vi "Get Queue Ref.vi"(6 "Command":T1=enum."Obtain", 8 "Error In":errorcluster, 11 "Call Chain Index (2)":i32=2) -> (0 "Error Out":errorcluster, 3 "Queue Out":T2)   [LabVIEW 2014, in "SLL QSM.lvlib"]
doc: "Create/Obtain/Delete Queue Reference based on the VI Instance Name. \n\nThe input to the call chain determines the VI for which the Queue Reference need to be obtained."
uses:
  SLL QSM.lvlib
  Typedefs/Queue Reference.ctl
  Typedefs/Queue Type.ctl
  Typedefs/Queue Reference Command.ctl
  Typedefs/Variant LUT Command.ctl
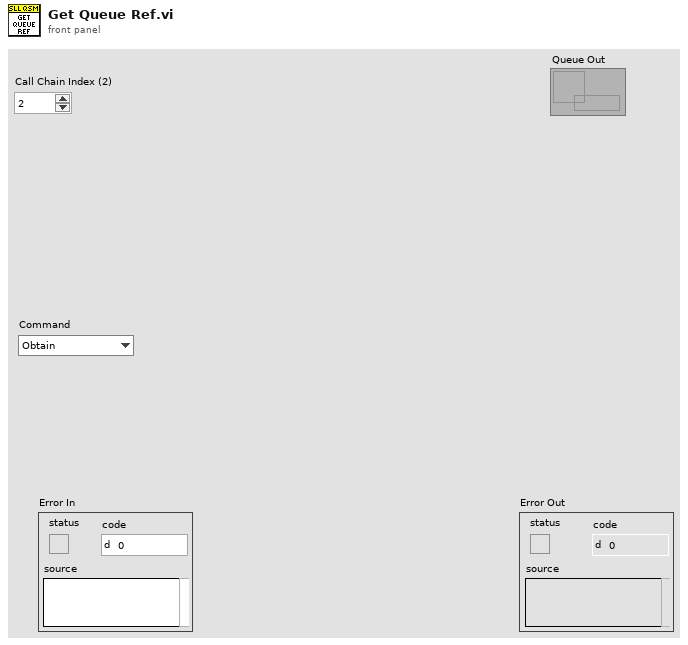
[diagram p1: front panel]
types:
  T1 = typedef "SLL QSM.lvlib/Queue Reference Command.ctl" = enum16{"Create", "Obtain", "Delete"}
  T2 = typedef "SLL QSM.lvlib/Queue Reference.ctl" = refnum<queue>
  T3 = typedef "SLL QSM.lvlib/Variant LUT Command.ctl" = enum16{"Get", "Set", "Delete"}
  T4 = typedef "SLL QSM.lvlib/Queue Type.ctl" = cluster{"State":string, "Data":variant}
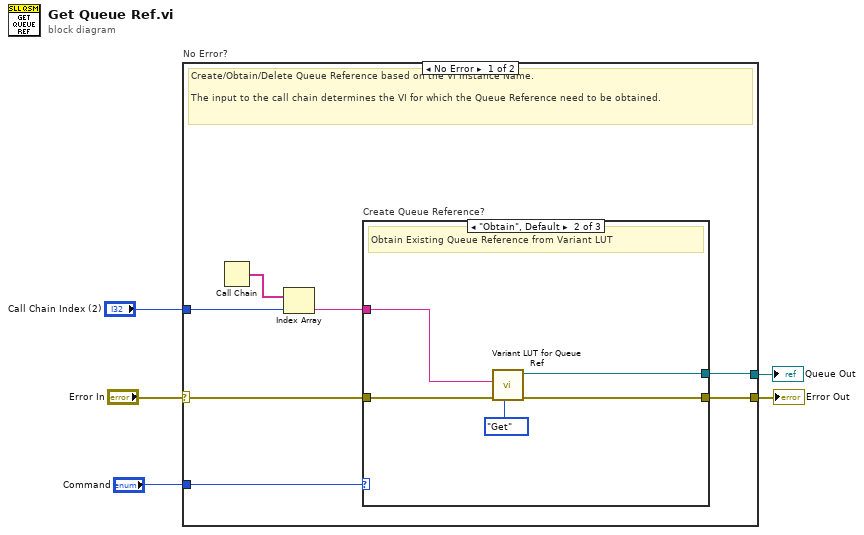
[diagram p0: block diagram]
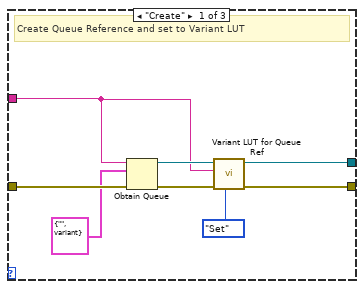
[diagram p2: hidden frame]
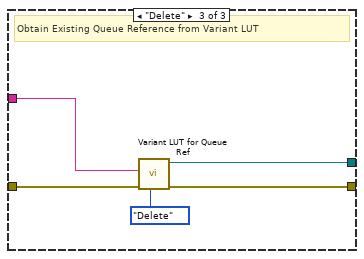
[diagram p3: hidden frame]
diagram:
  n1 = case "No Error?" shown="No Error" "Error In" {
    selector: "Error In" -> [w8 w31]
    tunnel: [w12 w31] -> w5
    tunnel: [w11 _] -> w3
    tunnel: "Call Chain Index (2)" -> [w9 _]
    tunnel: "Command" -> [w6 _]
    frame No Error {
      # "Create/Obtain/Delete Queue Reference based on the VI Instance Name. \n\nThe input to the call chain determines the VI for which the Queue Reference need to be obtained."
      n2 = Call Chain() -> (call chain=w10:string[])
      n3 = Index Array(array=w10, index=w9) -> (element=w7:string)
      n4 = case "Create Queue Reference?" shown="\"Obtain\", Default" w6 {
        tunnel: [w17 w23 w28] -> w12
        tunnel: [w15 w22 w27] -> w11
        tunnel: w8 -> [w20 w25 w30]
        tunnel: w7 -> [w13 w24 w29]
        frame "Create" {
          # "Create Queue Reference and set to Variant LUT"
          n5 = Obtain Queue(name (unnamed)=w13, element data type=T4 {"State"="", "Data"=variant} ("Queue Type"), error in (no error)=w20) -> (queue out=w16:refnum<queue>, error out=w18:errorcluster)  [unwired: 2 in, 1 out]
          n6 = call "Variant LUT for Queue Ref.vi"("Command"=Variant_LUT_Command."Set", "Error In"=w18, "Queue Name"=w13, "Queue Ref In"=w16) -> ("Error Out"=w17:errorcluster, "Queue Ref Out"=w15:T2)  [unwired: 6 in]
        }
        frame "Obtain", Default {
          # "Obtain Existing Queue Reference from Variant LUT"
          n7 = call "Variant LUT for Queue Ref.vi"("Command"=Variant_LUT_Command."Get", "Error In"=w25, "Queue Name"=w24) -> ("Error Out"=w23:errorcluster, "Queue Ref Out"=w22:T2)  [unwired: 7 in]
        }
        frame "Delete" {
          # "Obtain Existing Queue Reference from Variant LUT"
          n8 = call "Variant LUT for Queue Ref.vi"("Command"=Variant_LUT_Command."Delete", "Error In"=w30, "Queue Name"=w29) -> ("Error Out"=w28:errorcluster, "Queue Ref Out"=w27:T2)  [unwired: 7 in]
        }
      }
    }
    frame Error {
    }
  }
  "Error Out" <- w5
  "Queue Out" <- w3
